vi "Not A Refnum (TDMS).vi"(8 "error in (no error)":errorcluster, 11 "TDMS Log File in":refnum<class "TDMS Log File.lvclass">) -> (0 "error out":errorcluster, 2 "Not a Refnum?":bool, 3 "TDMS Log File out":refnum<class "TDMS Log File.lvclass">)   [LabVIEW 2012, in "Waveform Data Logger Engine.lvlib" / "TDMS Log File.lvclass"]
uses:
  TDMS Log File.lvclass
  TDMS Log File.lvclass/TDMS Log File.ctl
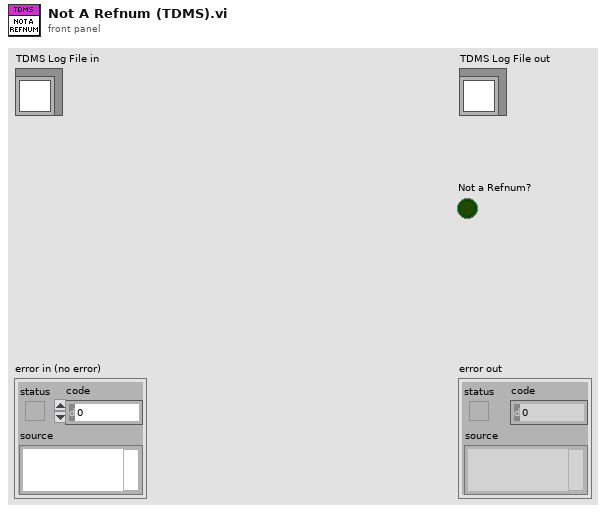
[diagram p1: front panel]
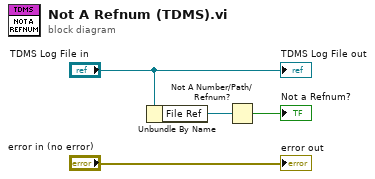
[diagram p0: block diagram]
diagram:
  n1 = Unbundle By Name("TDMS Log File in") -> ("File Ref"=w2:refnum<k34>)
  n2 = Not A Number/Path/Refnum?(number/path/refnum=w2) -> (NaN/Path/Refnum?=→"Not a Refnum?":bool)
  "error out" <- "error in (no error)"
  "TDMS Log File out" <- "TDMS Log File in"
